vi "Create CLI Script quitLabVIEW.vi"(8 "error in (no error)":errorcluster, 11 "PostBuildSupport in":refnum<class "PostBuildSupport.lvclass">) -> (0 "error out":errorcluster, 2 "command":string, 3 "PostBuildSupport out":refnum<class "PostBuildSupport.lvclass">)   [LabVIEW 2019, in "PostBuildSupport.lvclass"]
uses:
  PostBuildSupport.lvclass
  PostBuildSupport.lvclass/PostBuildSupport.ctl
  VIPM/VIPM.lvlib
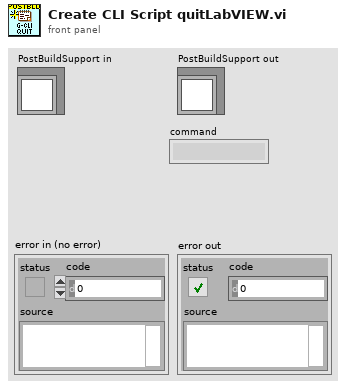
[diagram p1: front panel]
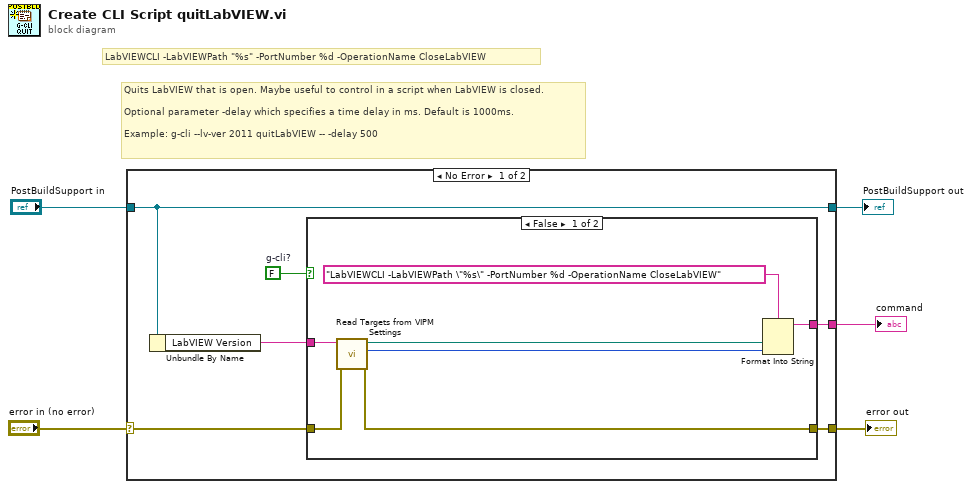
[diagram p0: block diagram]
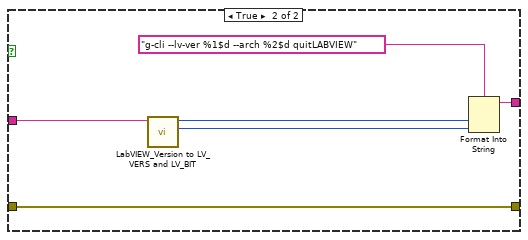
[diagram p2: hidden frame]
diagram:
  # "LabVIEWCLI -LabVIEWPath \"%s\" -PortNumber %d -OperationName CloseLabVIEW"
  # "Quits LabVIEW that is open. Maybe useful to control in a script when LabVIEW is closed.\n\nOptional parameter -delay which specifies a time delay in ms. Default is 1000ms.\n\nExample: g-cli --lv-ver 2011 quitLabVIEW -- -delay 500"
  n1 = case shown="No Error" "error in (no error)" {
    selector: "error in (no error)" -> [w7 w26]
    tunnel: "PostBuildSupport in" -> [w11 w25]
    tunnel: [w11 w25] -> w3
    tunnel: [w10 _] -> w2
    tunnel: [w6 w26] -> w1
    frame No Error {
      w9 = FALSE  # g-cli?
      n2 = Unbundle By Name(w11) -> ("LabVIEW Version"=w8:string)
      n3 = case shown="False" w9 {
        tunnel: [w18 w23] -> w10
        tunnel: w8 -> [w16 w20]
        tunnel: w7 -> [w15 w19]
        tunnel: [w14 w19] -> w6
        frame False {
          n4 = call "Read Targets from VIPM Settings.vi"("error in (no error)"=w15, "Version Filter"=w16) -> ("error out"=w14:errorcluster, "Port"=w12:i32, "Path"=w13:path)  [unwired: 6 in, 1 out]
          n5 = Format Into String(format string="LabVIEWCLI -LabVIEWPath \"%s\" -PortNumber %d -OperationName CloseLabVIEW", w13, w12) -> (resulting string=w18:string)  [unwired: 2 in, 1 out]
        }
        frame True {
          n6 = call "LabVIEW_Version to LV_VERS and LV_BIT.vi"("Package_LabVIEW_Version"=w20) -> ("LV_BIT"=w21:u32, "LV_VER"=w22:u32)  [unwired: 9 in]
          n7 = Format Into String(format string="g-cli --lv-ver %1$d --arch %2$d quitLABVIEW", w22, w21) -> (resulting string=w23:string)  [unwired: 2 in, 1 out]
        }
      }
    }
    frame Error {
    }
  }
  "error out" <- w1
  "PostBuildSupport out" <- w3
  "command" <- w2
